vi "FPGA_OffsetWithdrawSimulator.vi"() -> ()   [LabVIEW 2014]
uses:
  <vilib>/rvi/Emulation/niFpgaGetClockAttributes.vi
  <vilib>/rvi/Emulation/niFpgaSctlEmulationGetInTimedLoop.vi
  <vilib>/rvi/Emulation/niFpgaEmulationReportErrorSimple.vi
  <vilib>/rvi/Emulation/niFpgaCriticalErrorInLSC.vi
  <vilib>/rvi/interface/RandomDataEmulation/niFpgaRandomDataHandleErrors.vi
  <vilib>/rvi/DataTransferAndStorage/Container/XNode/niFpgaContainer.xnode
  <vilib>/rvi/interface/RandomDataEmulation/nirviRandomDataFpgaReadWriteTemplate.vi
panel:
  out "MaxZPos":i16(graph)
  out "PIZPos":i16
  out "PIZPosDia":i16(graph)
  in  "stop":bool
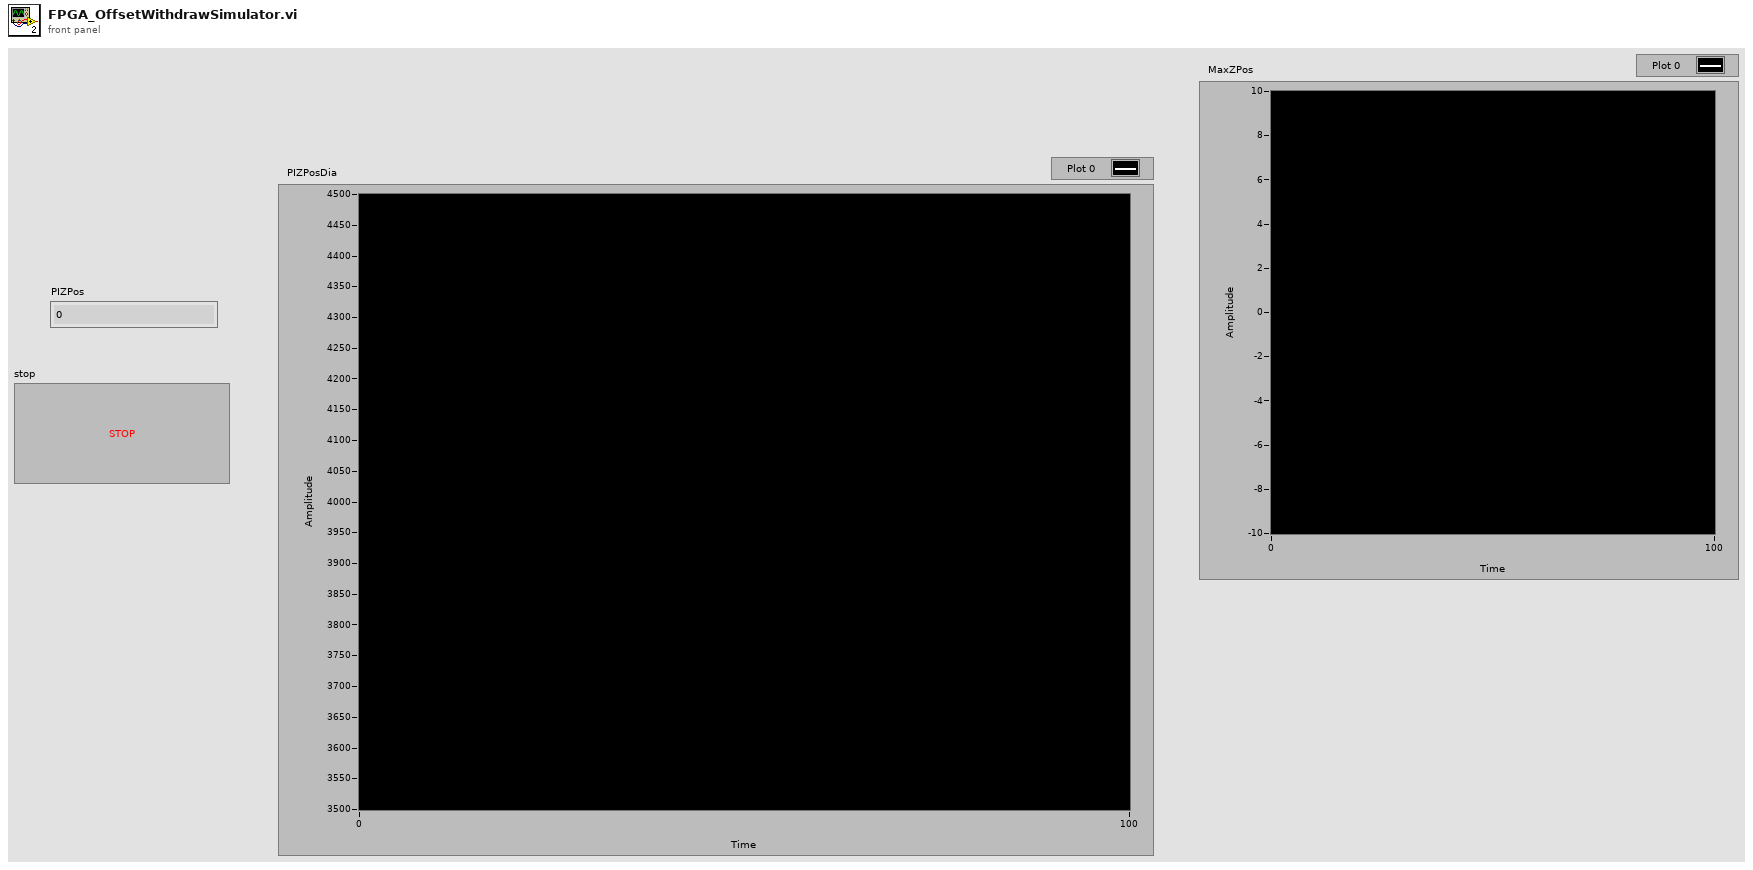
[diagram p1: front panel]
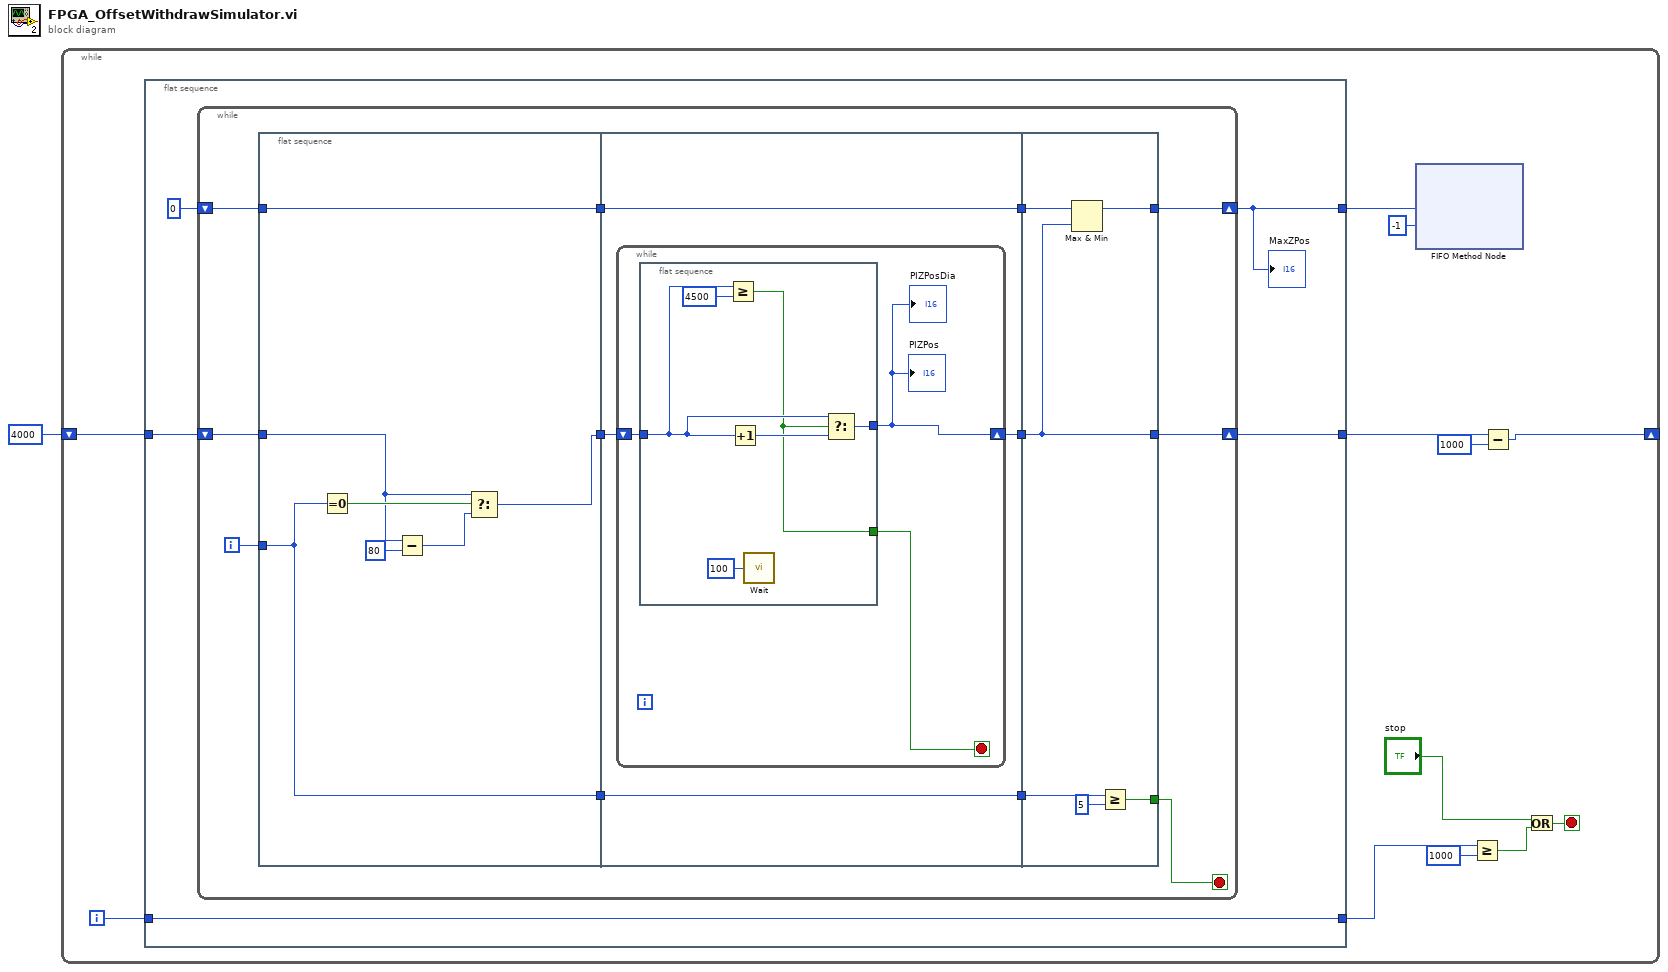
[diagram p0: block diagram]
diagram:
  n1 = while {
    shift-right: [w11] -> _
    shift-left: i16 4000 -> [w13]
    i -> [w10]
    stop <- w9 stop-if-true
    n2 = flat-sequence {
      tunnel: w13 -> [w18]
      tunnel: [w17] -> w4
      tunnel: w10 -> [w16]
      tunnel: [w16] -> w7
      tunnel: [w14] -> w2
      frame #0 {
        n3 = while {
          shift-right: [w27] -> w17
          shift-left: w18 -> [w28]
          shift-right: [w20] -> w14
          shift-left: i16 0 -> [w21]
          i -> [w26]
          stop <- w23 stop-if-true
          n4 = flat-sequence {
            tunnel: w28 -> [w34]
            tunnel: [w33] -> w30
            tunnel: w26 -> [w32]
            tunnel: [w32] -> w25
            tunnel: [w31] -> w22
            tunnel: w21 -> [w31]
            tunnel: w30 -> [w41]
            tunnel: [w40] -> w29
            tunnel: w25 -> [w39]
            tunnel: [w39] -> w24
            tunnel: w22 -> [w38]
            tunnel: [w38] -> w19
            tunnel: w29 -> [w51]
            tunnel: [w51] -> w27
            tunnel: w24 -> [w56]
            tunnel: [w55] -> w23
            tunnel: [w52] -> w20
            tunnel: w19 -> [w53]
            frame #0 {
              n5 = Equal To 0?(x=w32) -> (x = 0?=w37:bool)
              n6 = Subtract(x=w34, y=i16 80) -> (x-y=w35:i16)
              n7 = Select(t=w34, s=w37, f=w35) -> (s? t:f=w33:i16)
            }
            frame #1 {
              n8 = while {
                shift-right: [w42] -> w40
                shift-left: w41 -> [w44]
                stop <- w43 stop-if-true
                n9 = flat-sequence {
                  tunnel: w44 -> [w48]
                  tunnel: [w47] -> w42
                  tunnel: [w46] -> w43
                  frame #0 {
                    n10 = Greater Or Equal?(x=w48, y=i16 4500) -> (x >= y?=w46:bool)
                    n11 = Increment(x=w48) -> (x+1=w49:i16)
                    n12 = call "Wait"("Count(uSec)"=u32 100 ("Count(mSec)")) -> ()  [unwired: 1 out]
                    n13 = Select(t=w48, s=w46, f=w49) -> (s? t:f=w47:i16)
                  }
                }
                "PIZPosDia" <- w42
                "PIZPos" <- w42
              }
            }
            frame #2 {
              n14 = Max & Min(x=w53, y=w51) -> (max(x,y)=w52:i16)  [unwired: 1 out]
              n15 = Greater Or Equal?(x=w56, y=5) -> (x >= y?=w55:bool)
            }
          }
        }
        "MaxZPos" <- w14
      }
    }
    n16 = xnode ("FIFO Method Node")("Element"=w2, "Timeout"=-1) -> ()  [unwired: 1 in, 2 out]
    n17 = Greater Or Equal?(x=w7, y=1000) -> (x >= y?=w5:bool)
    n18 = Subtract(x=w4, y=i16 1000) -> (x-y=w11:i16)
    n19 = Or(x="stop", y=w5) -> (x .or. y?=w9:bool)
  }
